vi "rs3 start device.vi"(8 "error in":errorcluster, 11 "device":u32) -> (0 "error out":errorcluster, 3 "device":u64)   [LabVIEW 2023]
doc: "Start all enabled streams for this device."
uses:
  <vilib>/addons/RealSense/realsense-d.dll
panel:
  # "RS3 Start Device"
  # "(C) Intel Corp.,  AGJ"
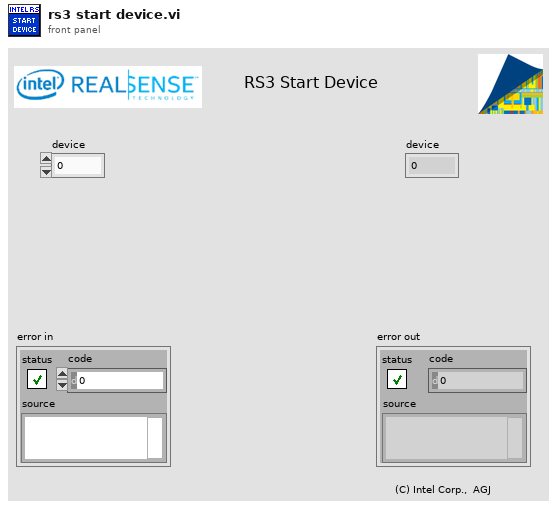
[diagram p1: front panel]
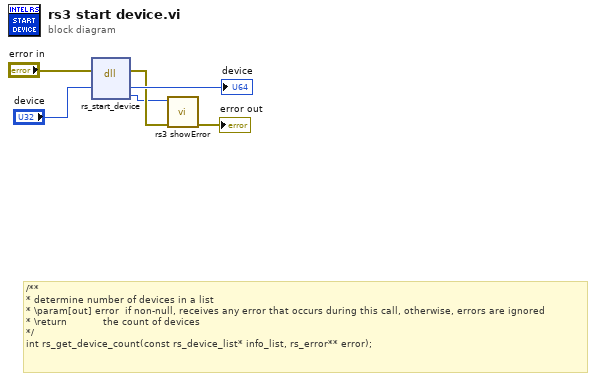
[diagram p0: block diagram]
diagram:
  # "/**\n* determine number of devices in a list\n* \\param[out] error  if non-null, receives any error that occurs during this call, otherwise, errors are ignored\n* \\return            the count of devices\n*/\nint rs_get_device_count(const rs_device_list* info_list, rs_error** error);"
  n1 = dll-call lib="C:/Program Files (x86)/National Instruments/LabVIEW 2017/vi.lib/addons/RealSense/realsense-d.dll" fn="rs_start_device"(error in="error in", "device"="device") -> (error out=w3:errorcluster, "device"=→"device":u32, "error"=w2:u64)  [unwired: 4 in, 1 out]
  n2 = call "rs3 showError.vi"("error in (no error)"=w3, "error"=w2) -> ("error out"=→"error out":errorcluster)  [unwired: 5 in, 4 out]
